vi "_OP_30.vi"(10 "OP_30 3":sgl[][](array[numeric]), 11 "OP_30 in":string[](array[string])) -> (2 "Cluster":T1, 3 "OP_30 out":T2)   [LabVIEW 2024]
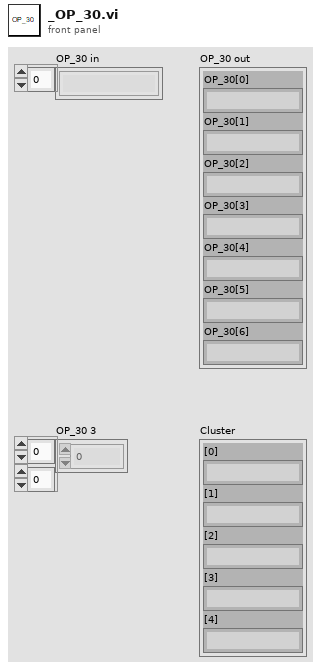
[diagram p1: front panel]
types:
  T1 = cluster{"[0]":string, "[1]":string, "[2]":string, "[3]":string, "[4]":string}
  T2 = cluster{"OP_30[0]":string, "OP_30[1]":string, "OP_30[2]":string, "OP_30[3]":string, "OP_30[4]":string, "OP_30[5]":string, "OP_30[6]":string}
  T3 = cluster{"OP_30 in[0]":string, "OP_30 in[1]":string, "OP_30 in[2]":string, "OP_30 in[3]":string, "OP_30 in[4]":string, "OP_30 in[5]":string, "OP_30 in[6]":string}
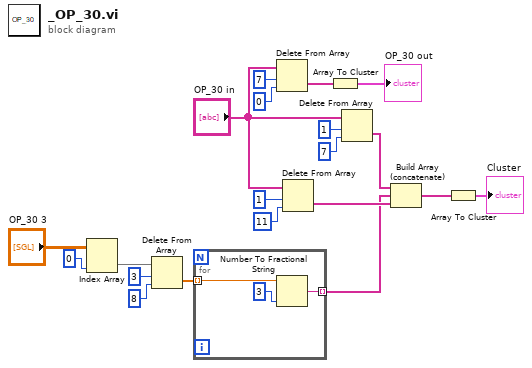
[diagram p0: block diagram]
diagram:
  n1 = Index Array(array="OP_30 3", index (col)=0 ("disabled index (col)")) -> (element=w7:sgl[])  [unwired: 1 in]
  n2 = Delete From Array(array=w7, length=3, index=8) -> (deleted portion=w6:sgl[])  [unwired: 1 out]
  n3 = for {
    tunnel: w6 -> [w22] mode=indexing
    tunnel: [w23] -> w12 mode=indexing
    n4 = Number To Fractional String(number=w22, precision (6)=i16 3) -> (F-format string=w23:string)  [unwired: 2 in]
  }
  n5 = Delete From Array(array="OP_30 in", length=7, index=0) -> (deleted portion=w19:string[])  [unwired: 1 out]
  n6 = Delete From Array(array="OP_30 in", length=1, index=11) -> (deleted portion=w13:string[])  [unwired: 1 out]
  n7 = Array To Cluster(array=w19) -> (cluster=→"OP_30 out":T3)
  n8 = Delete From Array(array="OP_30 in", length=1, index=7) -> (deleted portion=w18:string[])  [unwired: 1 out]
  n9 = Build Array (concatenate)(w18, w12, w13) -> (w14:string[])
  n10 = Array To Cluster(array=w14) -> (cluster=→"Cluster":T1)
